vi "Get Publish Data Events.vi"(11 "UserEvents in":refnum<class "User Events.lvclass">) -> (2 "Publish Data Events":T1, 3 "UserEvents out":refnum<class "User Events.lvclass">)   [LabVIEW 2016, in "User Events.lvclass"]
uses:
  User Events.lvclass
  Typedefs/Publish Data Events.ctl
  User Events.lvclass/User Events.ctl
  Typedefs/M1M3SupportEUI_TypeDefs.lvlib
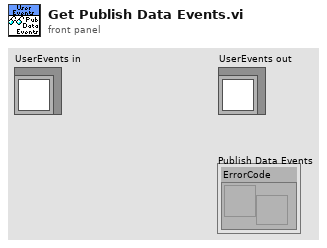
[diagram p1: front panel]
types:
  T1 = typedef "M1M3SupportEUI_TypeDefs.lvlib/Publish Data Events.ctl" = cluster{"ErrorCode":refnum<user-event>}
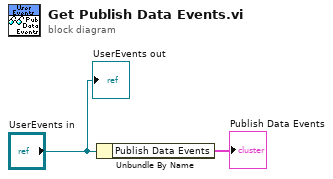
[diagram p0: block diagram]
diagram:
  n1 = Unbundle By Name("UserEvents in") -> ("Publish Data Events"=→"Publish Data Events":T1)
  "UserEvents out" <- "UserEvents in"
